vi "ValidDragDrop.vi"(8 "error in":errorcluster, 9 "Reorder":bool, 10 "drag over":string, 11 "Tree Ref in":refnum<vi>) -> (0 "Error Out":errorcluster, 1 "Accepted":bool, 2 "Drag":string, 3 "Tree Ref out":refnum<vi>, 4 "Moved Node":T1, 5 "Position":i32, 6 "Parent Node":T1, 7 "Parent":string)   [LabVIEW 2013, in "NISE_CEF_TreeControl.lvlib"]
doc: "This VI is used to see if a drag and drop operation is valid.\nThe drop shoudl be done in a node that accepts that kind of nodes."
uses:
  NISE_CEF_TreeControl.lvlib
  Node/NodeRef.ctl
  Node/NISE_CEF_Node.lvclass
  Node/ReadNodeClass.vi
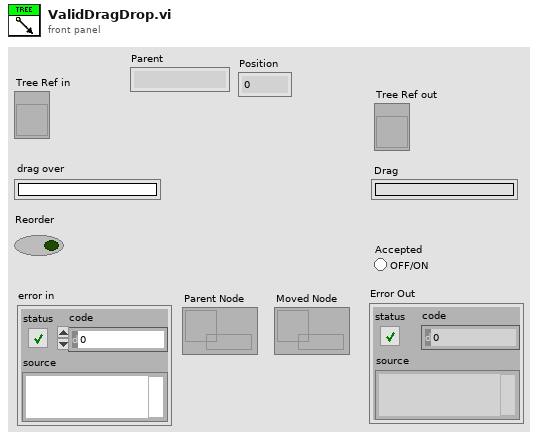
[diagram p1: front panel]
types:
  T1 = typedef "NISE_CEF_Node.lvclass/NodeRef.ctl" = refnum<data-value>
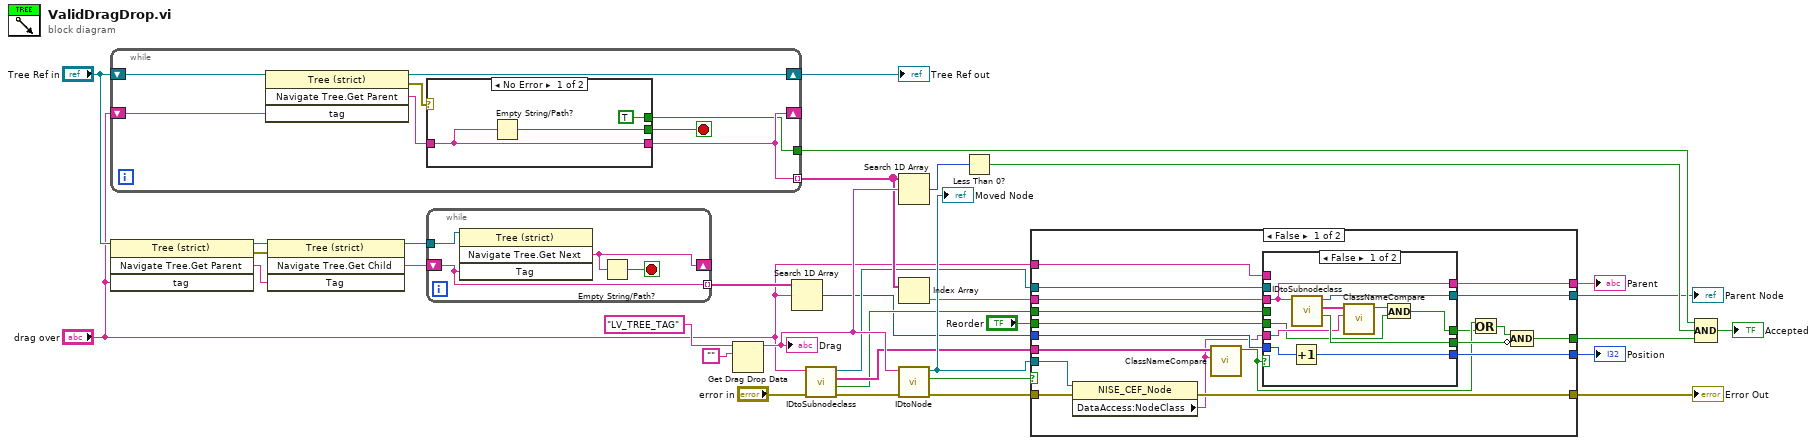
[diagram p0: block diagram]
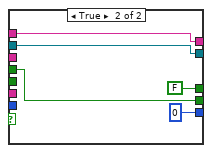
[diagram p2: hidden frame]
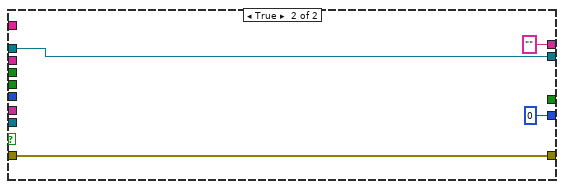
[diagram p3: hidden frame]
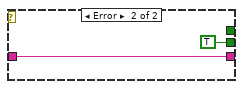
[diagram p4: hidden frame]
diagram:
  n1 = while {
    shift-right: [w36] -> _
    shift-left: "drag over" -> [w40]
    tunnel: [w36] -> w18 mode=indexing
    tunnel: [w35] -> w29
    shift-right: [w34] -> w30
    shift-left: "Tree Ref in" -> [w41]
    stop <- w39 stop-if-true
    n2 = invoke class="Tree (strict)" method="Navigate Tree.Get Parent"(reference=w41, "tag"=w40) -> (reference out=w34:refnum<vi>, error out=w38:errorcluster, "Navigate Tree:Get Parent"=w37:string)  [unwired: 2 in, 1 out]
    n3 = case shown="No Error" w38 {
      tunnel: [w42 TRUE] -> w39
      tunnel: w37 -> [w43 w45]
      tunnel: [w43 w45] -> w36
      tunnel: [TRUE _] -> w35
      frame No Error {
        n4 = Empty String/Path?(string/path=w43) -> (empty?=w42:bool)
      }
      frame Error {
      }
    }
  }
  "Tree Ref out" <- w30
  n5 = invoke class="Tree (strict)" method="Navigate Tree.Get Parent"(reference="Tree Ref in", "tag"="drag over") -> (reference out=w6:refnum<vi>, error out=w7:errorcluster, "Navigate Tree:Get Parent"=w8:string)  [unwired: 2 in, 1 out]
  n6 = invoke class="Tree (strict)" method="Navigate Tree.Get Child"(reference=w6, error in=w7, "Tag"=w8) -> (reference out=w5:refnum<vi>, "Navigate Tree:Get Child"=w4:string)  [unwired: 1 in, 2 out]
  n7 = while {
    shift-right: [w50] -> _
    shift-left: w4 -> [w47]
    tunnel: w5 -> [w48]
    tunnel: [w47] -> w3 mode=indexing
    stop <- w49 stop-if-true
    n8 = invoke class="Tree (strict)" method="Navigate Tree.Get Next"(reference=w48, "Tag"=w47) -> ("Navigate Tree:Get Next Item"=w50:string)  [unwired: 2 in, 3 out]
    n9 = Empty String/Path?(string/path=w50) -> (empty?=w49:bool)
  }
  n10 = Get Drag Drop Data(8:"", 9:"LV_TREE_TAG" ("data name")) -> (3:w26:string)  [unwired: 1 in, 1 out]
  "Drag" <- w26
  n11 = Search 1D Array(1D array=w3, element="drag over") -> (index of element=w1:i32)  [unwired: 1 in]
  n12 = call "IDtoSubnodeclass.vi"("error in (no error)"="error in", "Navigate Tree:Get Parent"="drag over") -> ("error out"=w11:errorcluster, "invalid Id"=w13:bool, "subnodes class"=w16:string[], "node ref"=w15:T1)  [unwired: 6 in]
  n13 = Search 1D Array(1D array=w18, element=w26) -> (index of element=w32:i32)  [unwired: 1 in]
  n14 = Index Array(array=w18) -> (element=w12:string)  [unwired: 1 in]
  n15 = call "IDtoNode.vi"("error in"=w11, "ID"=w26) -> ("error out"=w23:errorcluster, "invalid Id"=w24:bool, "node ref"=w25:T1)  [unwired: 7 in]
  "Moved Node" <- w25
  n16 = Less Than 0?(x=w32) -> (x < 0?=w28:bool)
  n17 = case shown="False" w24 {
    tunnel: w25 -> [w69 _]
    tunnel: w23 -> [w68 w88]
    tunnel: [w67 w88] -> w22
    tunnel: w16 -> [w64 _]
    tunnel: [w59 _] -> w21
    tunnel: [w66 w87] -> w19
    tunnel: w15 -> [w65 w87]
    tunnel: w1 -> [w63 _]
    tunnel: [w62 0] -> w14
    tunnel: w13 -> [w61 _]
    tunnel: w12 -> [w58 _]
    tunnel: [w53 "" ("drag over")] -> w10
    tunnel: "drag over" -> [w52 _]
    tunnel: "Reorder" -> [w51 _]
    frame False {
      n18 = property class="NISE_CEF_Node"(reference=w69, error in=w68) -> (error out=w67:errorcluster, "DataAccess:NodeClass"=w57:string)  [unwired: 1 out]
      n19 = call "ClassNameCompare.vi"("NodeClass"=w57, "classlist"=w64) -> ("match"=w56:bool)  [unwired: 9 in]
      n20 = case shown="False" w56 {
        tunnel: [w77 w84] -> w66
        tunnel: w65 -> [_ w84]
        tunnel: w63 -> [w79 _]
        tunnel: [w78 0] -> w62
        tunnel: w61 -> [_ w82]
        tunnel: [w76 w82] -> w60
        tunnel: w58 -> [w73 _]
        tunnel: w57 -> [w74 _]
        tunnel: [w70 FALSE ("match")] -> w55
        tunnel: [w73 w80] -> w53
        tunnel: w52 -> [_ w80]
        tunnel: w51 -> [w72 _]
        frame False {
          n21 = Increment(x=w79) -> (x+1=w78:i32)
          n22 = call "IDtoSubnodeclass.vi"("Navigate Tree:Get Parent"=w73) -> ("invalid Id"=w76:bool, "subnodes class"=w75:string[], "node ref"=w77:T1)  [unwired: 7 in, 1 out]
          n23 = call "ClassNameCompare.vi"("NodeClass"=w74, "classlist"=w75) -> ("match"=w71:bool)  [unwired: 9 in]
          n24 = And(x=w71, y=w72) -> (x .and. y?=w70:bool)
        }
        frame True {
        }
      }
      n25 = Or(x=w56, y=w55) -> (x .or. y?=w54:bool)
      n26 = Compound Arithmetic op=AND(w54, invert w60) -> (w59:bool)
    }
    frame True {
    }
  }
  "Error Out" <- w22
  "Parent Node" <- w19
  "Position" <- w14
  "Parent" <- w10
  n27 = Compound Arithmetic op=AND(w29, w28, w21) -> (→"Accepted":bool)
